vi "Actor Process.vi"(8 "error in":errorcluster, 11 "Actor Class":T1) -> (0 "error out":errorcluster)   [LabVIEW 2019]
uses:
  Actor Private Data.ctl
  <vilib>/LabVIEW Open Source Project/MQTT Client/Client class/Client.lvclass
  C:/Program Files (x86)/National Instruments/LabVIEW 2019/vi.lib/LabVIEW Open Source Project/MQTT Connection/MQTT_Base/Base Class/MQTT_Base.lvclass
  Actor Private Events -- cluster.ctl
  Payload -- cluster.ctl
  <vilib>/LabVIEW Open Source Project/MQTT Connection/MQTT_Base/Base Class/MQTT_Base.lvclass
panel:
  out "connected":bool
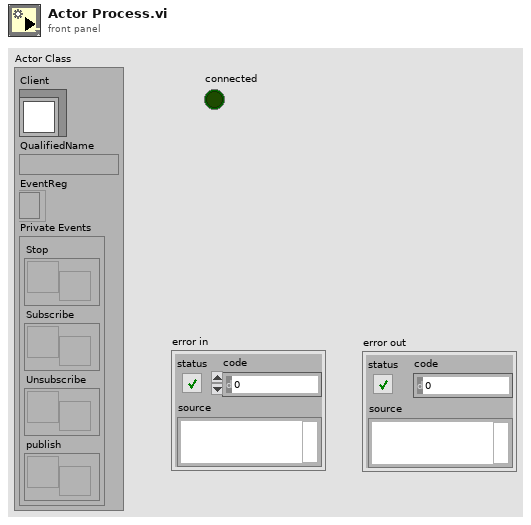
[diagram p1: front panel]
types:
  T1 = typedef "Actor Private Data.ctl" = cluster{"Client":refnum<class "Client.lvclass">, "QualifiedName":string, "EventReg":refnum<event-registration>, "Private Events":T2}
  T2 = typedef "Actor Private Events -- cluster.ctl" = cluster{"Stop":refnum<user-event>, "Subscribe":refnum<user-event>, "Unsubscribe":refnum<user-event>, "publish":refnum<user-event>}
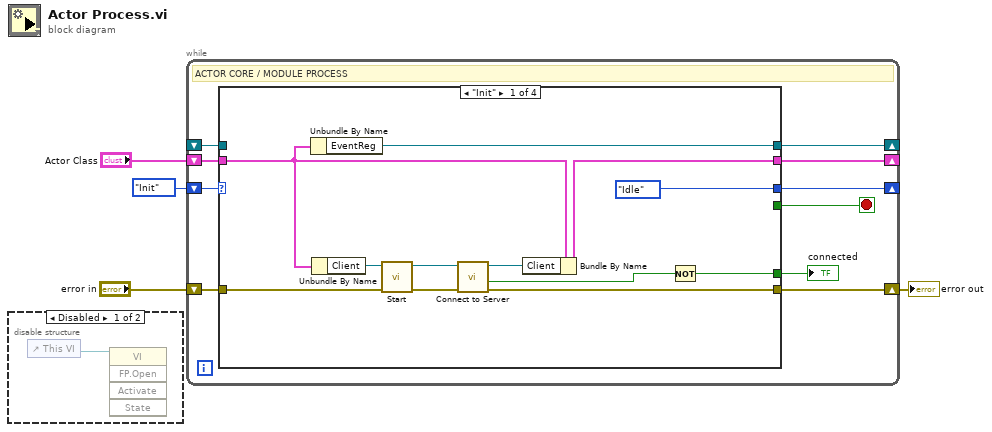
[diagram p0: block diagram]
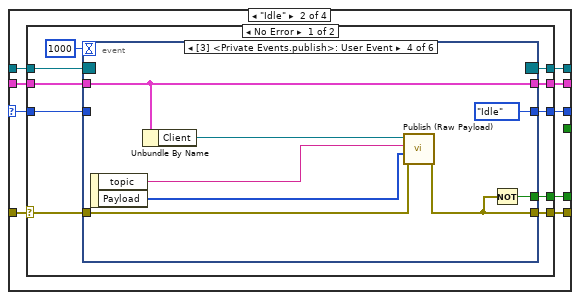
[diagram p3: hidden frame]
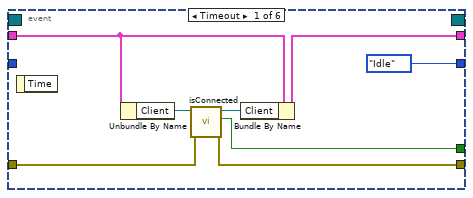
[diagram p4: hidden frame]
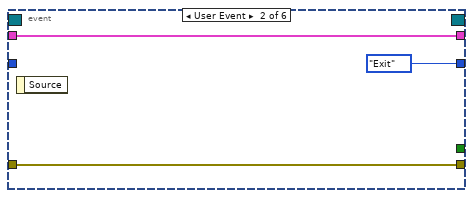
[diagram p5: hidden frame]
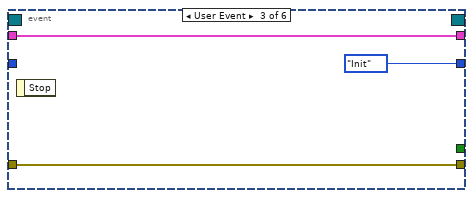
[diagram p6: hidden frame]
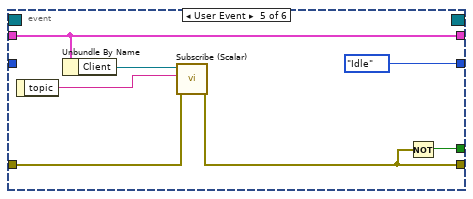
[diagram p7: hidden frame]
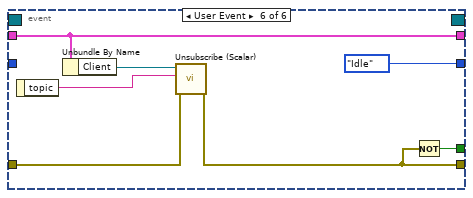
[diagram p8: hidden frame]
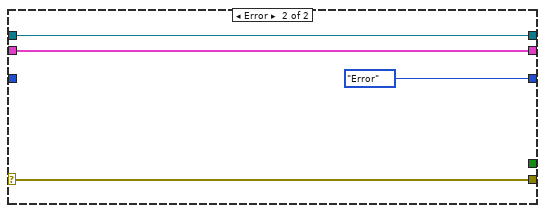
[diagram p9: hidden frame]
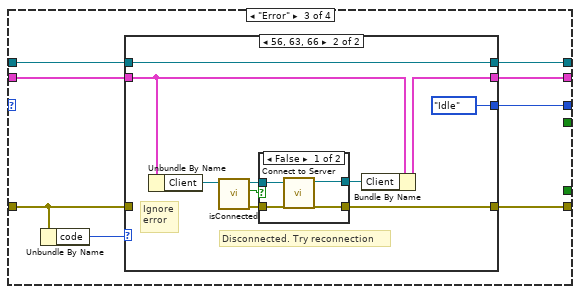
[diagram p10: hidden frame]
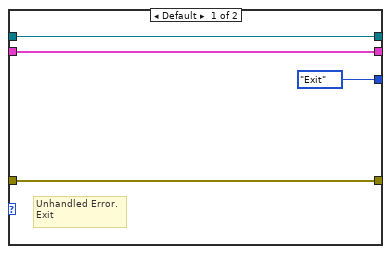
[diagram p11: hidden frame]
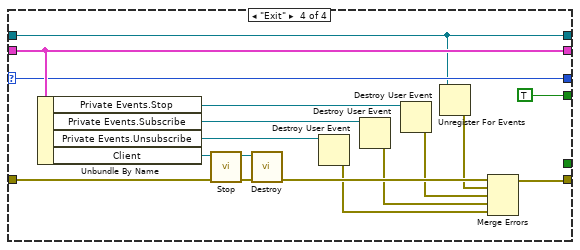
[diagram p13: hidden frame]
diagram:
  n1 = disable-structure shown="Disabled" {
    frame Disabled {
      n2 = control-ref of="This VI"() -> (w5:refnum<vi>)
      n3 = invoke class="VI" method="FP.Open"(reference=w5) -> ()  [unwired: 4 in, 5 out]
    }
    frame Enabled {
    }
  }
  n4 = while {
    shift-right: [w14] -> _
    shift-left: _ -> [w15]
    shift-right: [w13] -> w4
    shift-left: "error in" -> [w11]
    shift-right: [w7] -> _
    shift-left: enum16{"Init", "Idle", "Error", "Exit"}."Init" -> [w10]
    shift-right: [w9] -> _
    shift-left: "Actor Class" -> [w12]
    stop <- w8 stop-if-true
    # "ACTOR CORE / MODULE PROCESS"
    n5 = case shown="\"Init\"" w10 {
      selector: w10 -> [_ w32 _ w123]
      tunnel: w15 -> [_ w36 w87 w121]
      tunnel: [w25 w35 w88 w121] -> w14
      tunnel: [w20 w34 w92 w126] -> w13
      tunnel: w12 -> [w24 w33 w89 w125]
      tunnel: w11 -> [w22 w29 w94 w131]
      tunnel: [w26 w30 w90 w125] -> w9
      tunnel: [_ _ _ TRUE] -> w8
      tunnel: [enum16{"Init", "Idle", "Error", "Exit"}."Idle" w31 w91 w123] -> w7
      tunnel: [w16 w28 _ _] -> w6
      frame "Init" {
        n6 = Unbundle By Name(w24) -> ("EventReg"=w25:refnum<event-registration>)
        n7 = Unbundle By Name(w24) -> ("Client"=w23:refnum<class "Client.lvclass">)
        n8 = call <vilib>:"Start.vi"("error in (no error)"=w22, "MQTT_Base in"=w23) -> ("error out"=w21:errorcluster, "MQTT_Base out"=w19:refnum<class "Client.lvclass">)  [unwired: 7 in, 1 out]
        n9 = call <vilib>:"Connect to Server.vi"("error in (no error)"=w21, "Client in"=w19) -> ("error out"=w20:errorcluster, "timed out"=w17:bool, "Client out"=w18:refnum<class "Client.lvclass">)  [unwired: 6 in, 1 out]
        n10 = Bundle By Name(cluster=w24, "Client"=w18) -> (w26:T1)
        n11 = Not(x=w17) -> (.not. x?=w16:bool)
      }
      frame "Idle" {
        n12 = case shown="No Error" w29 {
          selector: w29 -> [w38 w83]
          tunnel: w36 -> [w46 w86]
          tunnel: [w45 w86] -> w35
          tunnel: [w44 w83] -> w34
          tunnel: w33 -> [w43 w85]
          tunnel: w32 -> [w41 _]
          tunnel: [w40 enum16{"Init", "Idle", "Error", "Exit"}."Error"] -> w31
          tunnel: [w39 w85] -> w30
          tunnel: [w37 _] -> w28
          frame No Error {
            n13 = event shown="[3] <Private Events.publish>: User Event" {
              selector: w46 -> [_ _ _ _ _ _]
              dyn-events: [_ _ _ _ _ _] -> w45
              timeout: 1000 -> [_ _ _ _ _ _]
              tunnel: w38 -> [w49 w57 w60 w66 w71 w78]
              tunnel: [w48 w57 w60 w63 w69 w76] -> w44
              tunnel: w43 -> [w51 w55 w58 w65 w74 w81]
              tunnel: w41 -> [_ _ _ _ _ _]
              tunnel: [enum16{"Init", "Idle", "Error", "Exit"}."Idle" enum16{"Init", "Idle", "Error", "Exit"}."Exit" enum16{"Init", "Idle", "Error", "Exit"}."Init" enum16{"Init", "Idle", "Error", "Exit"}."Idle" enum16{"Init", "Idle", "Error", "Exit"}."Idle" enum16{"Init", "Idle", "Error", "Exit"}."Idle"] -> w40
              tunnel: [w50 w55 w58 w65 w74 w81] -> w39
              tunnel: [w47 _ _ w64 w70 w77] -> w37
              event Timeout {
                n14 = event-data() -> ()  [unwired: 1 in, 1 out]
                n15 = Unbundle By Name(w51) -> ("Client"=w53:refnum<class "Client.lvclass">)
                n16 = call <vilib>:"isConnected.vi"("error in (no error)"=w49, "Client in"=w53) -> ("error out"=w48:errorcluster, "connected"=w47:bool, "Client out"=w52:refnum<class "Client.lvclass">)  [unwired: 7 in]
                n17 = Bundle By Name(cluster=w51, "Client"=w52) -> (w50:T1)
              }
              event User Event {
                n18 = event-data() -> ()  [unwired: 1 in, 1 out]
              }
              event User Event {
                n19 = event-data() -> ()  [unwired: 1 in, 1 out]
              }
              event User Event {
                n20 = event-data() -> ("topic"=w62:string, "Payload"=w61:u8[])  [unwired: 1 in]
                n21 = Unbundle By Name(w65) -> ("Client"=w67:refnum<class "Client.lvclass">)
                n22 = call <vilib>:"Publish (Raw Payload).vi"("error in (no error)"=w66, "Binary Payload"=w61, "Topic Name"=w62, "Client in"=w67) -> ("error out"=w63:errorcluster)  [unwired: 5 in, 2 out]
                n23 = Not(x=w63) -> (.not. x?=w64:bool)
              }
              event User Event {
                n24 = event-data() -> ("topic"=w73:string)  [unwired: 1 in]
                n25 = Unbundle By Name(w74) -> ("Client"=w72:refnum<class "Client.lvclass">)
                n26 = call <vilib>:"Subscribe (Scalar).vi"("error in (no error)"=w71, "Topic Filter"=w73, "Client in"=w72) -> ("error out"=w69:errorcluster)  [unwired: 6 in, 2 out]
                n27 = Not(x=w69) -> (.not. x?=w70:bool)
              }
              event User Event {
                n28 = event-data() -> ("topic"=w79:string)  [unwired: 1 in]
                n29 = Unbundle By Name(w81) -> ("Client"=w80:refnum<class "Client.lvclass">)
                n30 = call <vilib>:"Unsubscribe (Scalar).vi"("error in (no error)"=w78, "Topic Filter"=w79, "Client in"=w80) -> ("error out"=w76:errorcluster)  [unwired: 6 in, 2 out]
                n31 = Not(x=w76) -> (.not. x?=w77:bool)
              }
            }
          }
          frame Error {
          }
        }
      }
      frame "Error" {
        n32 = Unbundle By Name(w94) -> ("code"=w93:i32)
        n33 = case shown="56, 63, 66" w93 {
          tunnel: w94 -> [w97 _]
          tunnel: [w97 w105] -> w92
          tunnel: [enum16{"Init", "Idle", "Error", "Exit"}."Exit" enum16{"Init", "Idle", "Error", "Exit"}."Idle"] -> w91
          tunnel: [w95 w101] -> w90
          tunnel: w89 -> [w95 w100]
          tunnel: [w96 w99] -> w88
          tunnel: w87 -> [w96 w99]
          frame Default {
            # "Unhandled Error.\nExit"
          }
          frame 56, 63, 66 {
            # "Ignore\nerror"
            # "Disconnected. Try reconnection"
            n34 = Unbundle By Name(w100) -> ("Client"=w103:refnum<class "Client.lvclass">)
            n35 = call <vilib>:"isConnected.vi"("Client in"=w103) -> ("error out"=w107:errorcluster, "connected"=w106:bool, "Client out"=w108:refnum<class "Client.lvclass">)  [unwired: 8 in]
            n36 = case shown="False" w106 {
              tunnel: w108 -> [w112 w114]
              tunnel: w107 -> [w111 w113]
              tunnel: [w110 w114] -> w102
              tunnel: [w109 w113] -> w105
              frame False {
                n37 = call <vilib>:"Connect to Server.vi"("error in (no error)"=w111, "Client in"=w112) -> ("error out"=w109:errorcluster, "Client out"=w110:refnum<class "Client.lvclass">)  [unwired: 6 in, 2 out]
              }
              frame True {
              }
            }
            n38 = Bundle By Name(cluster=w100, "Client"=w102) -> (w101:T1)
          }
        }
      }
      frame "Exit" {
        n39 = Unbundle By Name(w125) -> ("Private Events.Stop"=w130:refnum<user-event>, "Private Events.Subscribe"=w119:refnum<user-event>, "Private Events.Unsubscribe"=w116:refnum<user-event>, "Client"=w120:refnum<class "Client.lvclass">)
        n40 = call <vilib>:"Stop.vi"("error in (no error)"=w131, "MQTT_Base in"=w120) -> ("error out"=w128:errorcluster, "MQTT_Base out"=w129:refnum<class "Client.lvclass">)  [unwired: 7 in, 1 out]
        n41 = call <vilib>:"Destroy.vi"("error in (no error)"=w128, "MQTT_Base in"=w129) -> ("error out"=w127:errorcluster)  [unwired: 8 in, 1 out]
        n42 = Destroy User Event(user event=w116) -> (error out=w115:errorcluster)  [unwired: 1 in]
        n43 = Destroy User Event(user event=w119) -> (error out=w117:errorcluster)  [unwired: 1 in]
        n44 = Destroy User Event(user event=w130) -> (error out=w118:errorcluster)  [unwired: 1 in]
        n45 = Unregister For Events(event registration refnum=w121) -> (error out=w122:errorcluster)  [unwired: 1 in]
        n46 = Merge Errors(w127, w122, w118, w117, w115) -> (w126:errorcluster)
      }
    }
    "connected" <- w6
  }
  "error out" <- w4
